vi "Read ctl.vi"(8 "error in (no error)":errorcluster, 11 "Update TEC PID in":refnum<class "Update TEC Multipliers.lvclass">=refnum) -> (0 "error out":errorcluster, 2 "ctl":cluster{"P":dbl, "I":dbl, "D":dbl}, 3 "Update TEC PID out":refnum<class "Update TEC Multipliers.lvclass">)   [LabVIEW 2014, in "Update TEC Multipliers.lvclass"]
uses:
  Update TEC Multipliers.lvclass
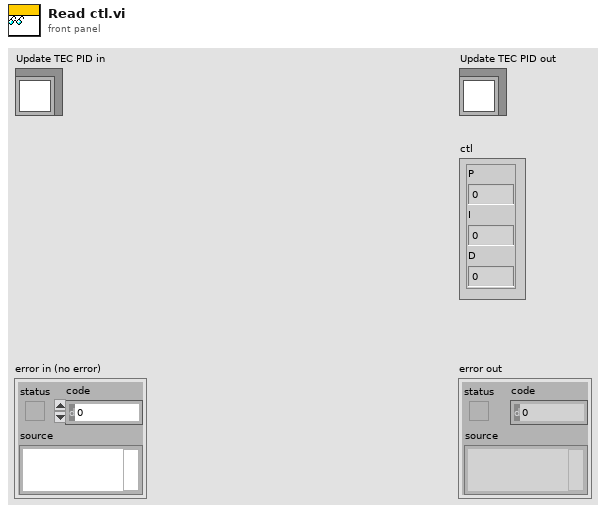
[diagram p1: front panel]
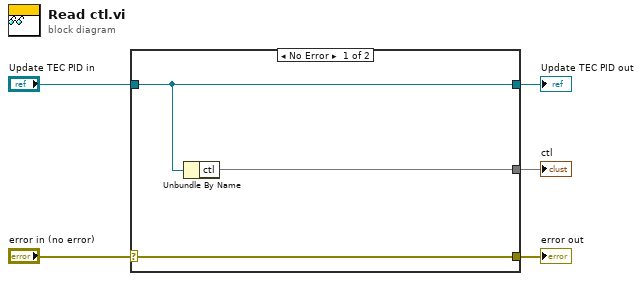
[diagram p0: block diagram]
diagram:
  n1 = case shown="No Error" "error in (no error)" {
    selector: "error in (no error)" -> [w8 w9]
    tunnel: [w8 w9] -> w4
    tunnel: [w7 w10] -> w2
    tunnel: "Update TEC PID in" -> [w7 w10]
    tunnel: [w6 _] -> w1
    frame No Error {
      n2 = Unbundle By Name(w7) -> ("ctl"=w6)
    }
    frame Error {
    }
  }
  "error out" <- w4
  "Update TEC PID out" <- w2
  "ctl" <- w1
